vi "LWXPS_SetJogVelocity.vi"(0 "XPS Reference IN":refnum<k24>, 5 "Velocity X":dbl, 7 "Velocity Y":dbl, 9 "Joystick Ack Timeout":i32, 11 "LabVIEW error IN":errorcluster) -> (4 "XPS Reference OUT":refnum<k24>, 6 "Returned error code":i32, 8 "XPS Error String":string, 15 "LabVIEW error OUT":errorcluster)   [LabVIEW 2014]
uses:
  D:/XPSQ8_LabView_Library/Development/Source/Dll/Newport.XPS.CommandInterface.dll
  Dll/Newport.XPS.CommandInterface.dll
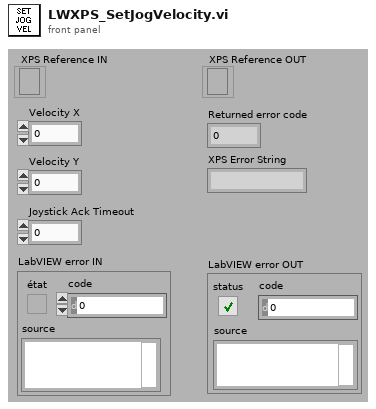
[diagram p1: front panel]
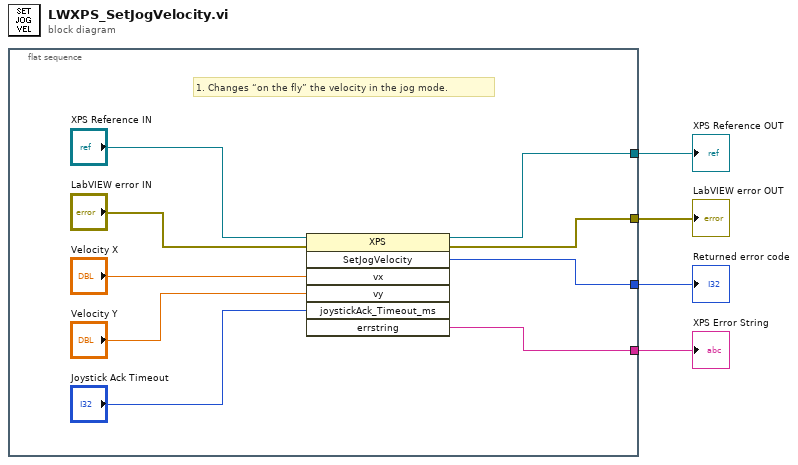
[diagram p0: block diagram]
diagram:
  n1 = flat-sequence {
    tunnel: [w12] -> w4
    tunnel: [w11] -> w3
    tunnel: [w5] -> w2
    tunnel: [w6] -> w1
    frame #0 {
      # "1. Changes “on the fly” the velocity in the jog mode."
      n2 = invoke class="XPS" method="SetJogVelocity"(reference="XPS Reference IN", error in="LabVIEW error IN", "vx"="Velocity X", "vy"="Velocity Y", "joystickAck_Timeout_ms"="Joystick Ack Timeout") -> (reference out=w12:refnum<k24>, error out=w11:errorcluster, "SetJogVelocity"=w6:i32, "errstring"=w5:string)  [unwired: 2 in, 3 out]
    }
  }
  "XPS Reference OUT" <- w4
  "LabVIEW error OUT" <- w3
  "XPS Error String" <- w2
  "Returned error code" <- w1
